vi "HISW-ProcessPAQsample.vi"(8 "error in (no error)":errorcluster, 10 "PAQdatagram IN":T1 {"data" format="%.2f"; "status" format="%08x"}, 11 "HISW in":refnum<class "HISW.lvclass">) -> (0 "error out":errorcluster, 3 "HISW out":refnum<class "HISW.lvclass">)   [LabVIEW 2020, in "Sgraph_lib_V1.lvlib" / "HISW.lvclass"]
uses:
  HISW.lvclass
  C:/Sgraph/source/AVPP/AVPP.lvclass
  controls/typedef_PAQdatagram.ctl
  AVPP/AVPP.lvclass
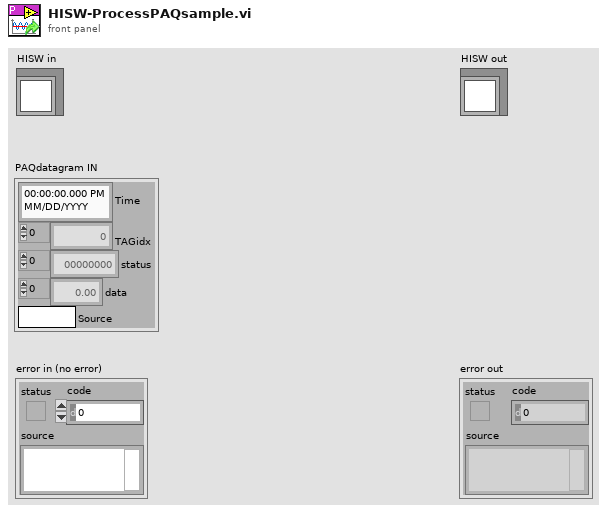
[diagram p1: front panel]
types:
  T1 = typedef "typedef_PAQdatagram.ctl" = cluster{"Time":timestamp, "TAGidx":i32[], "status":u32[], "data":dbl[], "Source":string}
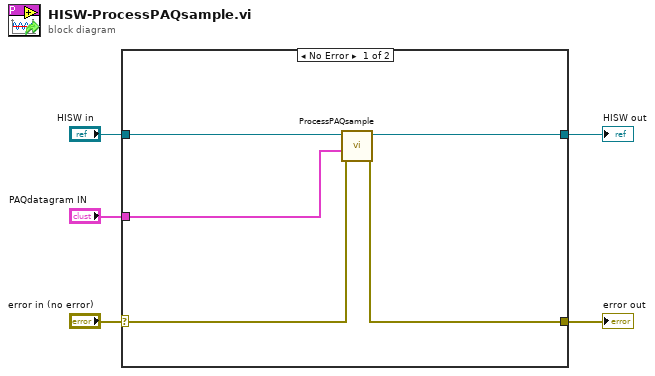
[diagram p0: block diagram]
diagram:
  n1 = case shown="No Error" "error in (no error)" {
    selector: "error in (no error)" -> [w10 w12]
    tunnel: [w9 w12] -> w4
    tunnel: [w6 w11] -> w2
    tunnel: "HISW in" -> [w7 w11]
    tunnel: "PAQdatagram IN" -> [w8 _]
    frame No Error {
      n2 = call "ProcessPAQsample.vi"("error in (no error)"=w10, "PAQdatagram IN"=w8, "AVPP in"=w7) -> ("error out"=w9:errorcluster, "AVPP out"=w6:refnum<class "HISW.lvclass">)  [unwired: 7 in]
    }
    frame Error {
    }
  }
  "error out" <- w4
  "HISW out" <- w2
